vi "main.vi"() -> ()   [LabVIEW 2016]
panel:
  in  "Tab Control":T1(tab)
  in  "Resistencia":bool
  in  "Capacidade":bool
  in  "Carga":bool
  in  "stop":bool
  in  "Inicio3":bool
  in  "VISA":refnum<visa-resource-name>="GPIB::05::INSTR"
  in  "Voltage Limit":dbl format="%.4f"
  in  "Current Limit":dbl format="%.4f"
  in  "Output On (T)":bool=TRUE
  out "Output Voltage":dbl format="%.4f"
  out "Output Current":dbl format="%.4f"
  out "error out":errorcluster
  out "Waveform Chart Voltage":dbl(graph)
  in  "Inicio1":bool
  in  "Inicio2":bool
  # "MENU"
  # "Desenvolvido por William Rocha"
  # "CARGA"
  # "Desenvolvido por William Rocha"
  # "Right-Click to\nexplain error"
  # "ENSAIO DE CAPACIDADE"
  # "Desenvolvido por William Rocha"
  # "ENSAIO DE RESISTÊNCIA CC"
  # "Desenvolvido por William Rocha"
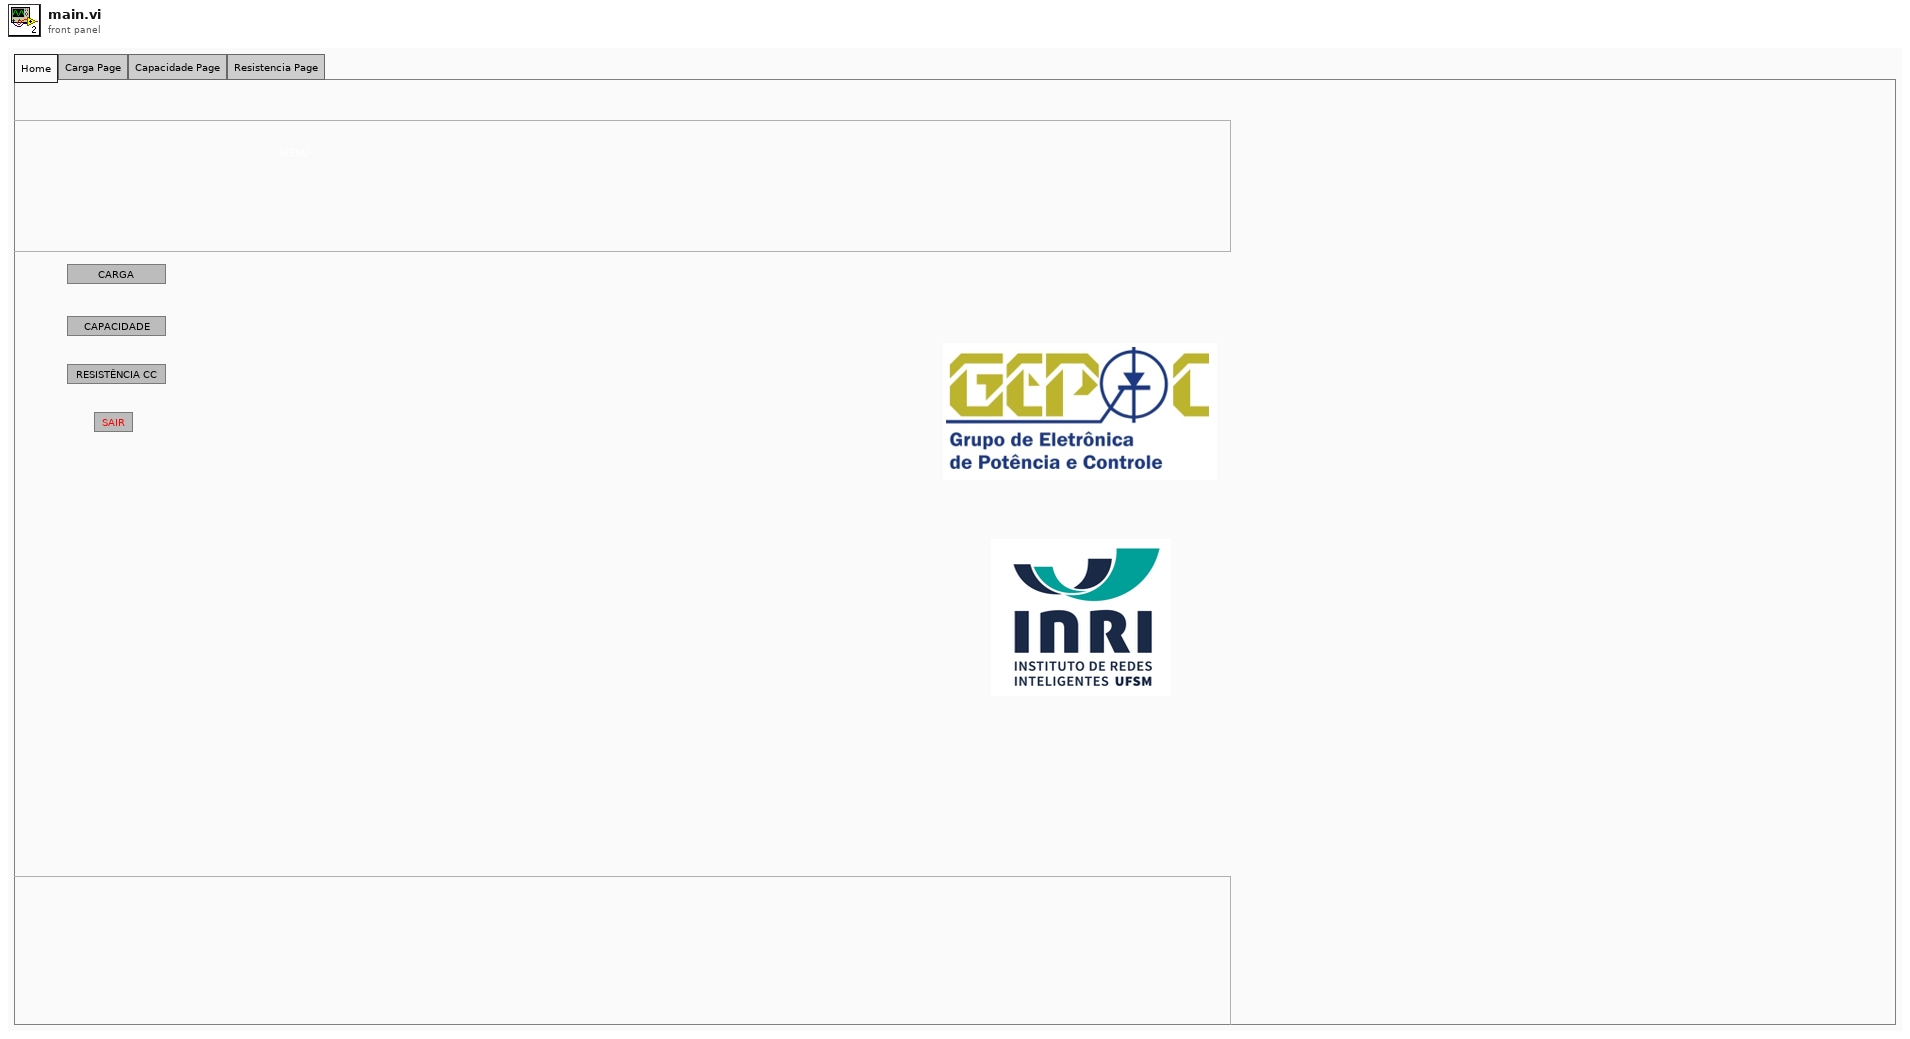
[diagram p1: front panel]
types:
  T1 = enum32{"Home", "Carga Page", "Capacidade Page", "Resistencia Page"}
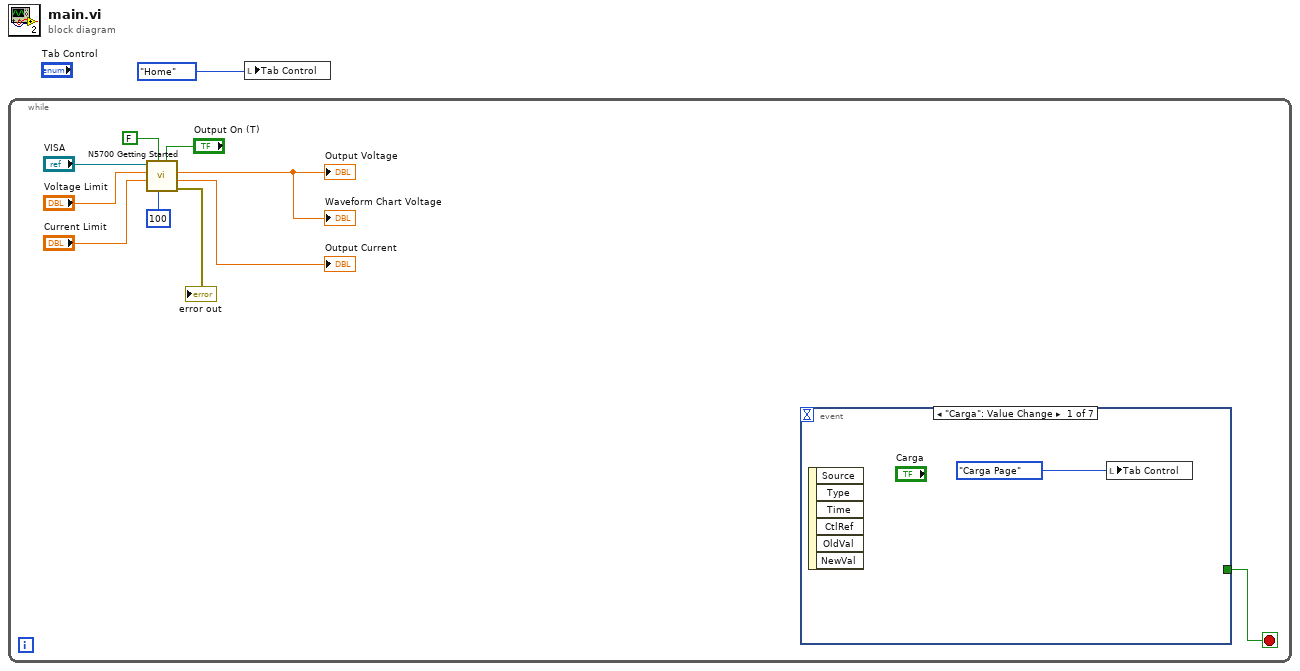
[diagram p0: block diagram]
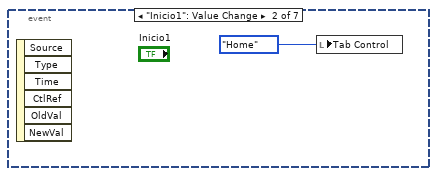
[diagram p2: hidden frame]
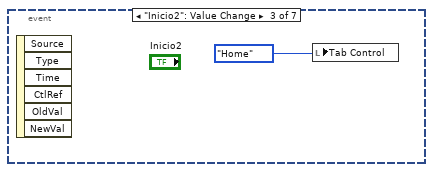
[diagram p3: hidden frame]
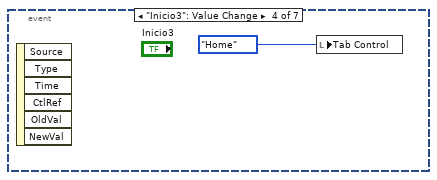
[diagram p4: hidden frame]
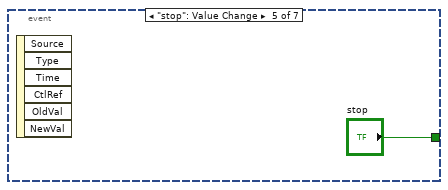
[diagram p5: hidden frame]
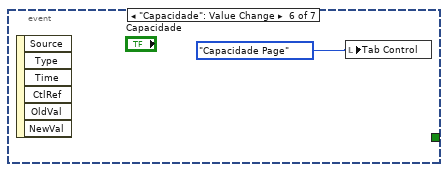
[diagram p6: hidden frame]
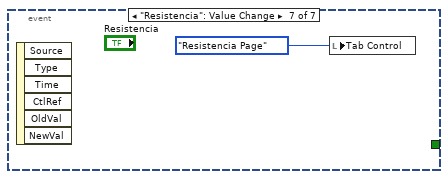
[diagram p7: hidden frame]
diagram:
  n1 = while {
    stop <- w11 stop-if-true
    n2 = call <instrlib>:"N5700 Getting Started.vi"("Output On (T)"="Output On (T)", "Settle (0 mS)"=u32 100, "Reset (F)"=FALSE, "Current Limit"="Current Limit", "Voltage Limit"="Voltage Limit", "VISA"="VISA") -> ("error out"=→"error out":errorcluster, "Output Current"=→"Output Current":dbl, "Output Voltage"=→"Output Voltage" →"Waveform Chart Voltage":dbl)  [unwired: 2 in, 1 out]
    n3 = event shown="[0] \"Carga\": Value Change" {
      selector: _ -> [_ _ _ _ _ _ _]
      dyn-events: _ -> [_ _ _ _ _ _ _]
      timeout: _ -> [_ _ _ _ _ _ _]
      tunnel: [_ _ _ _ "stop" _ _] -> w11
      event "Carga": Value Change {
        n4 = event-data() -> ()  [unwired: 1 in, 6 out]
        n5 = local write "Tab Control"(T1."Carga Page" ("Tab Control")) -> ()
      }
      event "Inicio1": Value Change {
        n6 = event-data() -> ()  [unwired: 1 in, 6 out]
        n7 = local write "Tab Control"(T1."Home" ("Tab Control")) -> ()
      }
      event "Inicio2": Value Change {
        n8 = event-data() -> ()  [unwired: 1 in, 6 out]
        n9 = local write "Tab Control"(T1."Home" ("Tab Control")) -> ()
      }
      event "Inicio3": Value Change {
        n10 = event-data() -> ()  [unwired: 1 in, 6 out]
        n11 = local write "Tab Control"(T1."Home" ("Tab Control")) -> ()
      }
      event "stop": Value Change {
        n12 = event-data() -> ()  [unwired: 1 in, 6 out]
      }
      event "Capacidade": Value Change {
        n13 = event-data() -> ()  [unwired: 1 in, 6 out]
        n14 = local write "Tab Control"(T1."Capacidade Page" ("Tab Control")) -> ()
      }
      event "Resistencia": Value Change {
        n15 = event-data() -> ()  [unwired: 1 in, 6 out]
        n16 = local write "Tab Control"(T1."Resistencia Page" ("Tab Control")) -> ()
      }
    }
  }
  n17 = local write "Tab Control"(T1."Home" ("Tab Control")) -> ()
